vi "Vision Processing.vi"(4 "error in (no error)":errorcluster) -> ()   [LabVIEW 2016]
doc: "This VI runs in parallel to other tasks. It gets images from the camera, processes them for color or shape and use that information to affect robot behavior."
uses:
  <vilib>/Rock Robotics/WPI/Camera/WPI_CameraImageSize.ctl
  Camera Settings.ctl
  38 Video Mode.ctl
  Robot Global Data.vi
  <vilib>/Rock Robotics/WPI/Camera/WPI_CameraWhite Balance Values.ctl
  <vilib>/Rock Robotics/WPI/Camera/WPI_CameraExposure Values.ctl
  <vilib>/Rock Robotics/WPI/Camera/WPI_CameraFrameRate.ctl
panel:
  out "Image":T1(plugin-control)
  in  "error in (no error) 2":errorcluster
  out "Array 2":errorcluster[](array[cluster])
  in  "Image Size 2":T2=enum."320x240"
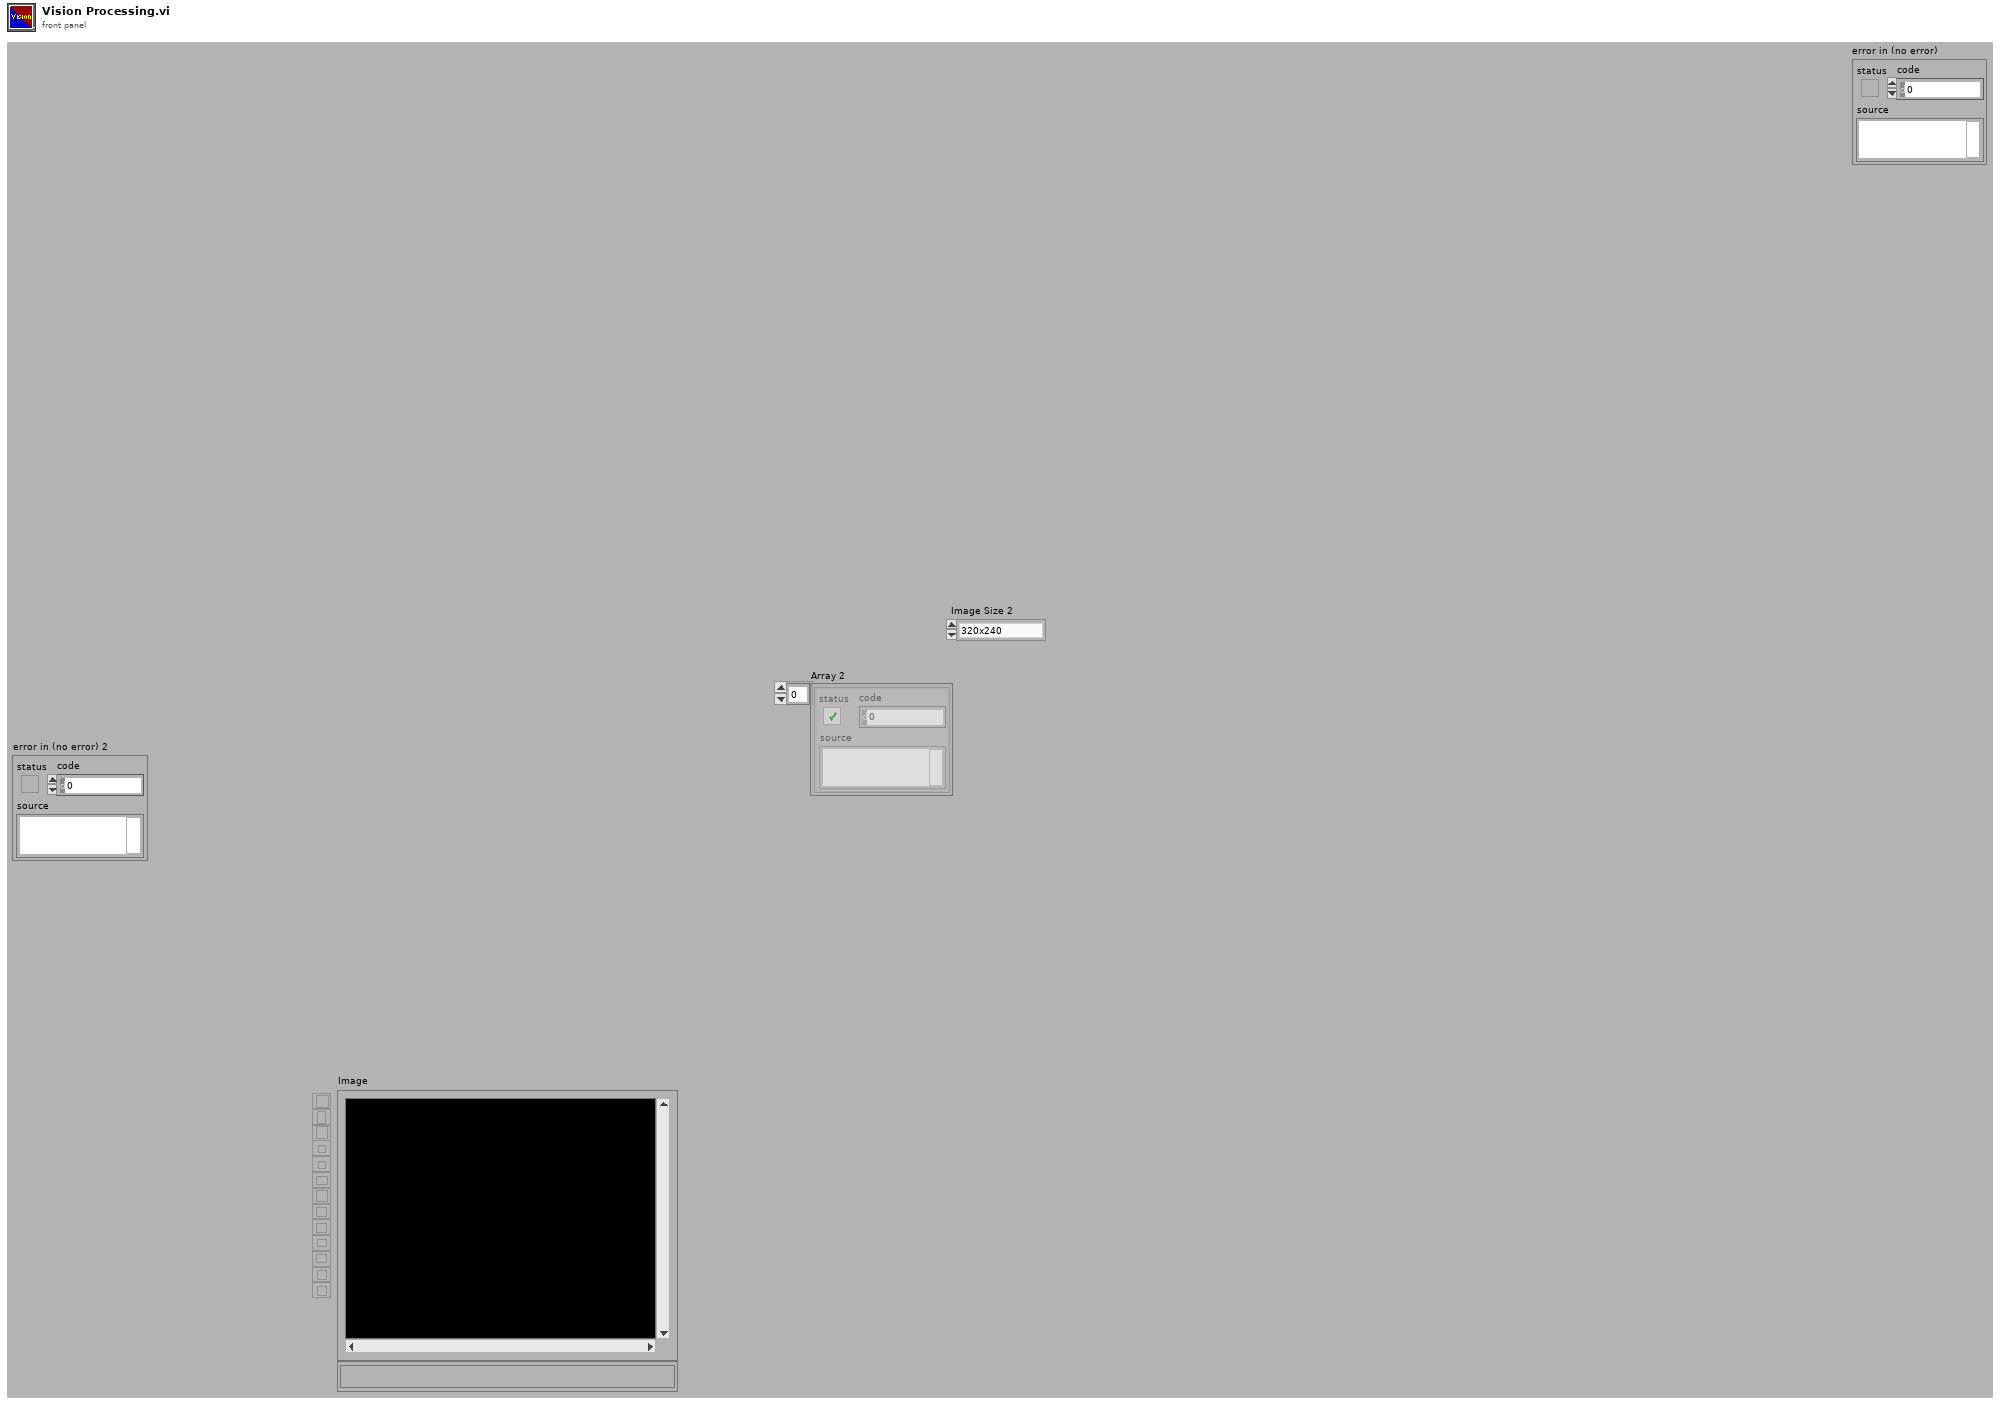
[diagram p1: front panel]
types:
  T1 = typedef "IMAQ Image.ctl" = refnum<image>
  T2 = typedef "WPI_CameraImageSize.ctl" = enum16{"640x480", "320x240", "160x120", "Custom"}
  T3 = typedef "Camera Settings.ctl" = cluster{"VideoMode":T4, "Brightness":i64, "Sharpness":i64, "White Balance":i64, "Saturation":i64, "Exposure":i64}
  T4 = typedef "38 Video Mode.ctl" = u32
  T5 = typedef "WPI_CameraFrameRate.ctl" = u32
  T6 = typedef "WPI_CameraExposure Values.ctl" = enum16{"Auto", "Flicker-free 50 Hz", "Flicker-free 60 Hz", "Hold current", "Custom"}
  T7 = typedef "WPI_CameraWhite Balance Values.ctl" = enum16{"Auto", "Fixed indoor", "Fixed outdoor 1", "Fixed outdoor 2", "Fixed fluorescent 1", "Fixed fluorescent 2", "Hold current", "Custom"}
  T8 = typedef "Image Type" = u32
  T9 = typedef "WPI_CameraDevRef.ctl" = cluster{"Camera Address":string, "CameraStatus":errorcluster}
  T10 = typedef "TCP Port Control.ctl" = cluster{"TCP Ports":cluster{"listener ID":refnum<k5>, "port":u16}[], "semaphore":T11, "occurrence":refnum<k4>, "Listener":refnum<data-value>}
  T11 = typedef "Semaphore RefNum" = refnum<k1>
  T12 = typedef "IMAQdx.ctl" = refnum<k21>
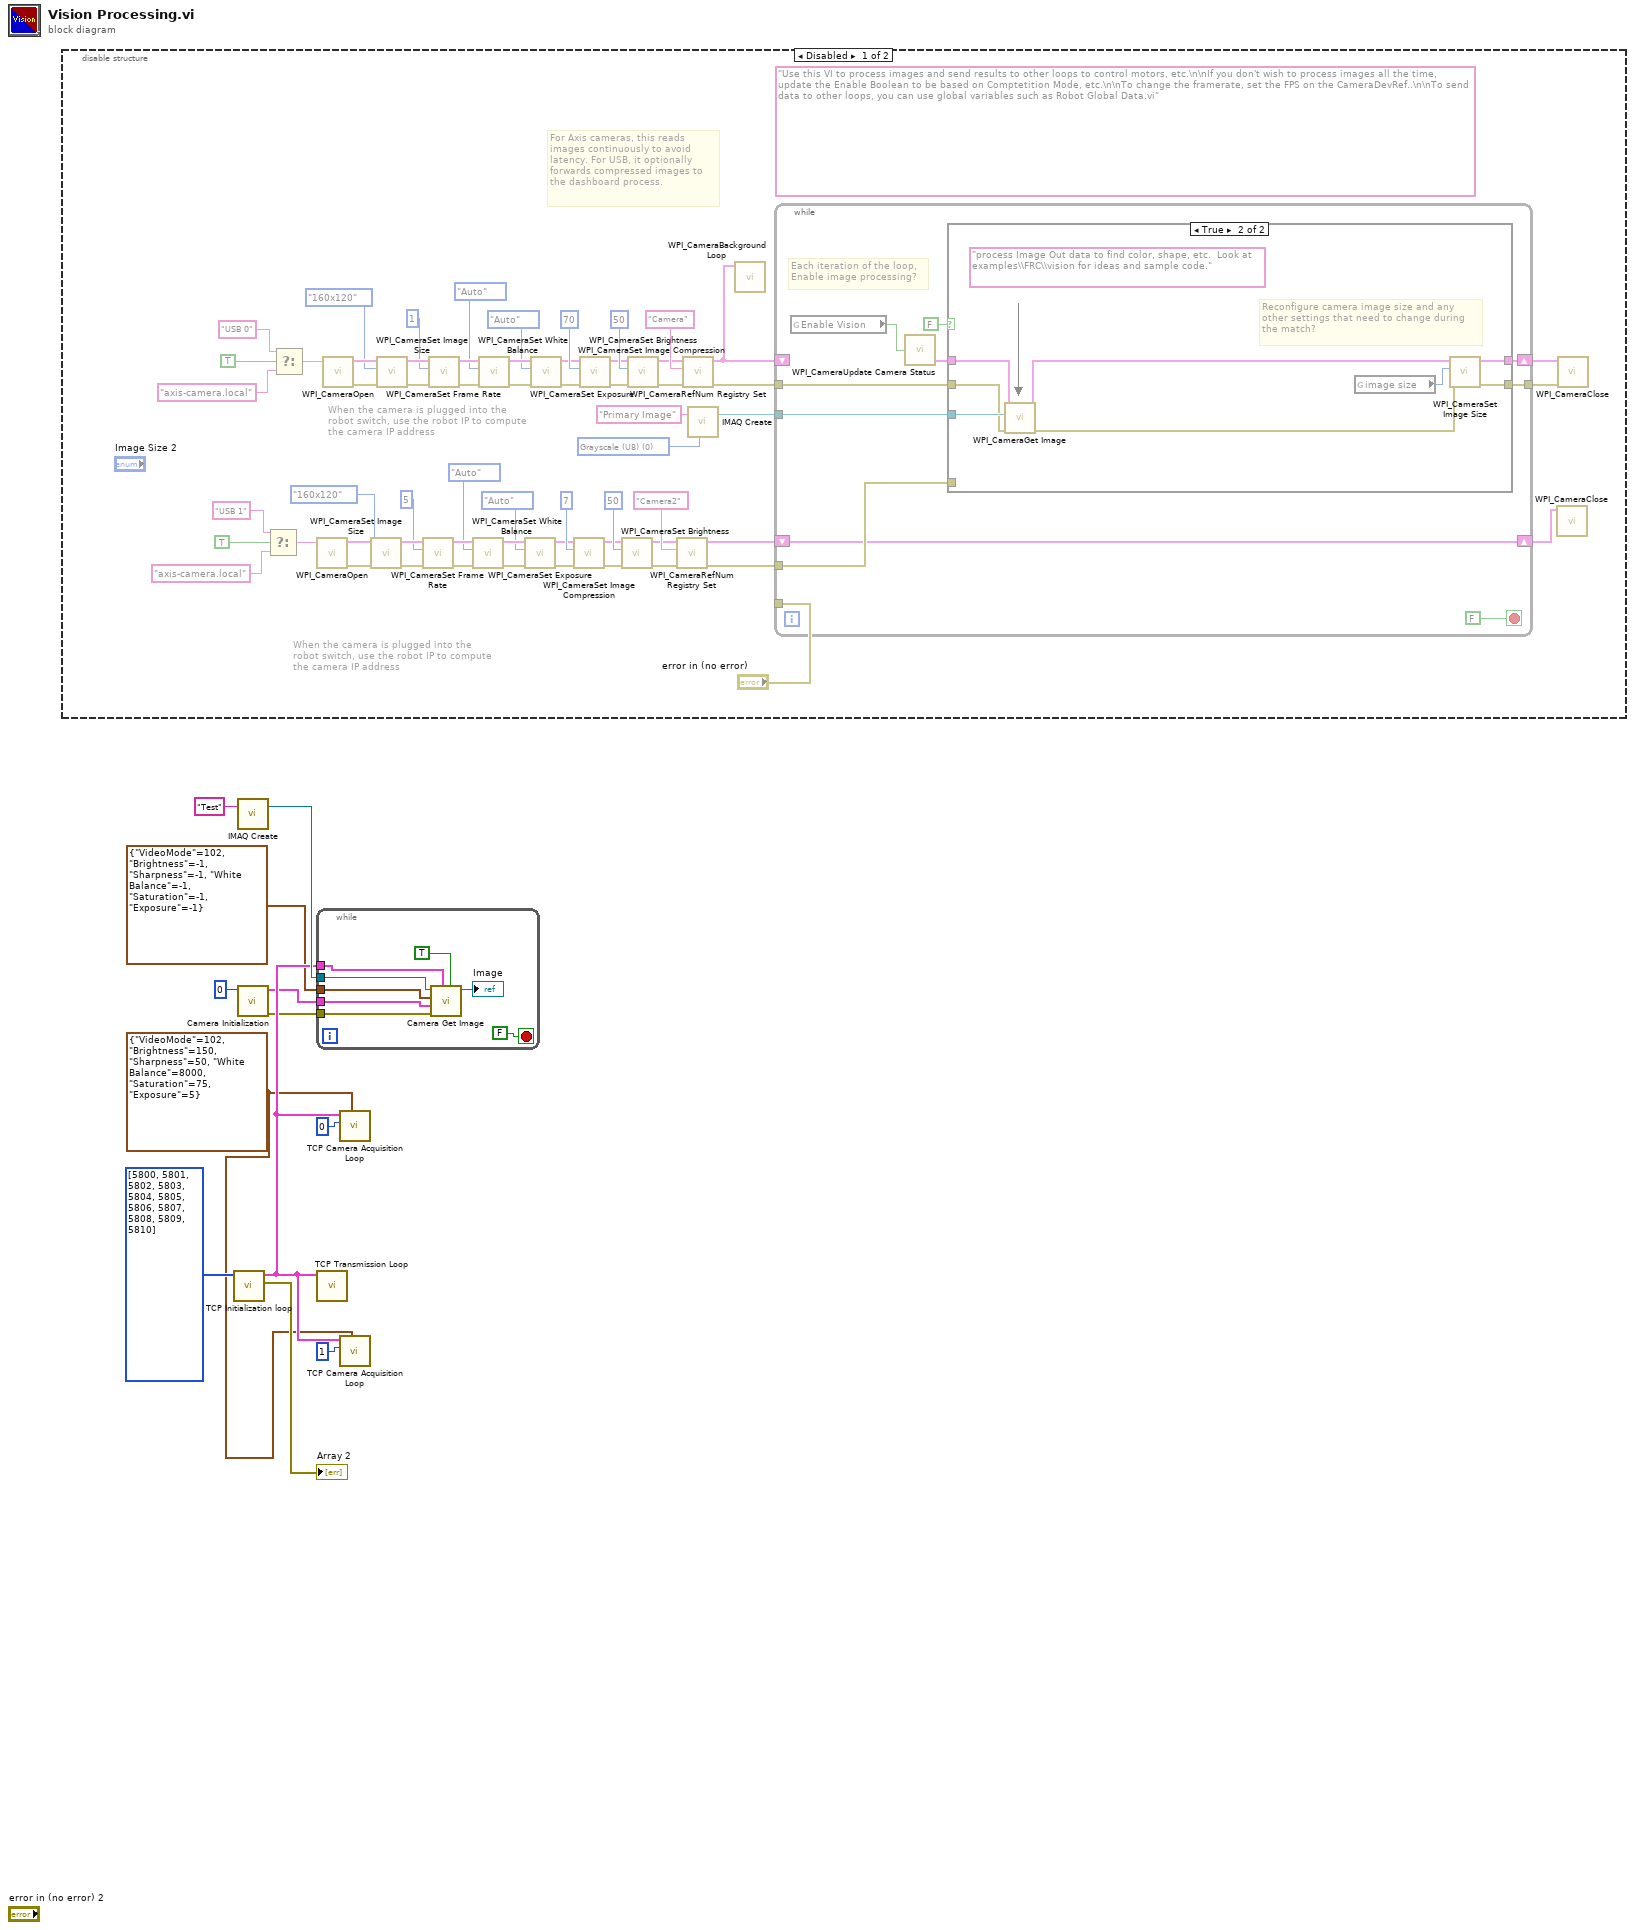
[diagram p0: block diagram]
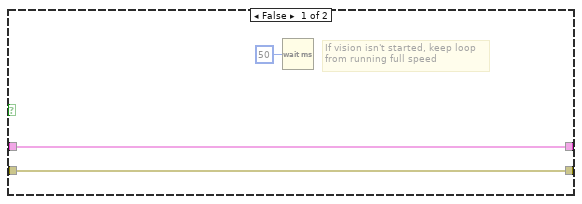
[diagram p2: hidden frame]
diagram:
  w1 = T3 {"VideoMode"=102, "Brightness"=150, "Sharpness"=50, "White Balance"=8000, "Saturation"=75, "Exposure"=5} ("Camera Controls")
  n1 = disable-structure shown="Disabled" {
    frame Disabled {
      (unwired) "Use this VI to process images and send results to other loops to control motors, etc.\n\nIf you don't wish to process images all the time, update the Enable Boolean to be based on Comptetition Mode, etc.\n\nTo change the framerate, set the FPS on the CameraDevRef..\n\nTo send data to other loops, you can use global variables such as Robot Global Data.vi"
      w73 = T8 0 items=["Grayscale (U8)", "Grayscale (I16)", "Grayscale (SGL)", "Complex (CSG)", "RGB (U32)", "HSL (U32)", "RGB (U64)"] ("Image Type")
      # "When the camera is plugged into the\nrobot switch, use the robot IP to compute\nthe camera IP address"
      # "When the camera is plugged into the\nrobot switch, use the robot IP to compute\nthe camera IP address"
      # "For Axis cameras, this reads\nimages continuously to avoid\nlatency. For USB, it optionally\nforwards compressed images to\nthe dashboard process."
      n2 = Select(t="USB 1" ("format string"), s=TRUE ("dot notation? (F)"), f="axis-camera.local" ("format string")) -> (s? t:f=w20:string)
      n3 = Select(t="USB 0" ("format string"), s=TRUE ("dot notation? (F)"), f="axis-camera.local" ("format string")) -> (s? t:f=w44:string)
      n4 = call <vilib>:"WPI_CameraOpen.vi"("Camera Address"=w20) -> ("error out"=w33:errorcluster, "CameraDevRef"=w34:T9)  [unwired: 1 in, 8 out]
      n5 = call <vilib>:"WPI_CameraOpen.vi"("Camera Address"=w44) -> ("error out"=w61:errorcluster, "CameraDevRef"=w62:T9)  [unwired: 1 in, 8 out]
      n6 = call <vilib>:"WPI_CameraSet Image Size.vi"("error in (no error)"=w33, "Image Size"=WPI_CameraImageSize."160x120", "CameraDevRef"=w34) -> ("error out"=w32:errorcluster, "CameraDevRef Out"=w35:T9)  [unwired: 1 in, 6 out]
      n7 = call <vilib>:"WPI_CameraSet Image Size.vi"("error in (no error)"=w61, "Image Size"=WPI_CameraImageSize."160x120", "CameraDevRef"=w62) -> ("error out"=w60:errorcluster, "CameraDevRef Out"=w63:T9)  [unwired: 1 in, 6 out]
      n8 = call <vilib>:"WPI_CameraSet Frame Rate.vi"("error in (no error)"=w32, "Frame Rate (fps)"=T5 5, "CameraDevRef"=w35) -> ("error out"=w31:errorcluster, "CameraDevRef Out"=w37:T9)  [unwired: 7 out]
      n9 = call <vilib>:"WPI_CameraSet Frame Rate.vi"("error in (no error)"=w60, "Frame Rate (fps)"=T5 1, "CameraDevRef"=w63) -> ("error out"=w59:errorcluster, "CameraDevRef Out"=w65:T9)  [unwired: 7 out]
      n10 = call <vilib>:"WPI_CameraSet White Balance.vi"("error in (no error)"=w31, "White Balance"=WPI_CameraWhite_Balance_Values."Auto", "CameraDevRef"=w37) -> ("error out"=w30:errorcluster, "CameraDevRef Out"=w36:T9)  [unwired: 1 in, 6 out]
      n11 = call <vilib>:"WPI_CameraSet White Balance.vi"("error in (no error)"=w59, "White Balance"=WPI_CameraWhite_Balance_Values."Auto", "CameraDevRef"=w65) -> ("error out"=w58:errorcluster, "CameraDevRef Out"=w64:T9)  [unwired: 1 in, 6 out]
      n12 = call <vilib>:"WPI_CameraSet Exposure.vi"("error in (no error)"=w30, "Exposure"=WPI_CameraExposure_Values."Auto", "CameraDevRef"=w36) -> ("error out"=w29:errorcluster, "CameraDevRef Out"=w39:T9)  [unwired: 1 in, 6 out]
      n13 = call <vilib>:"WPI_CameraSet Exposure.vi"("error in (no error)"=w58, "Exposure"=WPI_CameraExposure_Values."Auto", "CameraDevRef"=w64) -> ("error out"=w57:errorcluster, "CameraDevRef Out"=w67:T9)  [unwired: 1 in, 6 out]
      n14 = call <vilib>:"WPI_CameraSet Image Compression.vi"("error in (no error)"=w29, "Compression"=7, "CameraDevRef"=w39) -> ("error out"=w28:errorcluster, "CameraDevRef Out"=w38:T9)  [unwired: 7 out]
      n15 = call <vilib>:"WPI_CameraSet Image Compression.vi"("error in (no error)"=w57, "Compression"=70, "CameraDevRef"=w67) -> ("error out"=w56:errorcluster, "CameraDevRef Out"=w66:T9)  [unwired: 7 out]
      n16 = call <vilib>:"WPI_CameraSet Brightness.vi"("error in (no error)"=w28, "Brightness"=50, "CameraDevRef"=w38) -> ("error out"=w26:errorcluster, "CameraDevRef Out"=w27:T9)  [unwired: 7 out]
      n17 = call <vilib>:"WPI_CameraSet Brightness.vi"("error in (no error)"=w56, "Brightness"=50, "CameraDevRef"=w66) -> ("error out"=w54:errorcluster, "CameraDevRef Out"=w55:T9)  [unwired: 7 out]
      n18 = call <vilib>:"WPI_CameraRefNum Registry Set.vi"("error in (no error)"=w26, "refnum name"="Camera2", "CameraDevRef"=w27) -> ("error out"=w14:errorcluster, "CameraDevRef"=w13:T9)  [unwired: 1 in, 6 out]
      n19 = call <vilib>:"WPI_CameraRefNum Registry Set.vi"("error in (no error)"=w54, "refnum name"="Camera", "CameraDevRef"=w55) -> ("error out"=w16:errorcluster, "CameraDevRef"=w50:T9)  [unwired: 1 in, 6 out]
      n20 = call "IMAQ Create"("Image Name"="Primary Image", "Image Type"=w73) -> ("New Image"=w71:T1)  [unwired: 2 in, 2 out]
      n21 = call <vilib>:"WPI_CameraBackground Loop.vi"("CameraDevRef"=w50) -> ()  [unwired: 11 in]
      n22 = while {
        shift-right: [w82] -> w48
        shift-left: w50 -> [_]
        tunnel: w71 -> [w81]
        tunnel: "error in (no error)" -> [_]
        tunnel: w16 -> [w78]
        tunnel: [w77] -> w15
        tunnel: w14 -> [w76]
        shift-right: [w74] -> w18
        shift-left: w13 -> [w74]
        stop <- FALSE stop-if-true
        # "Each iteration of the loop,\nEnable image processing?"
        n23 = global read "Robot Global Data.vi" "Enable Vision"() -> (w79:bool)
        n24 = call <vilib>:"WPI_CameraUpdate Camera Status.vi"("Enable Vision"=w79) -> ("CameraDevRef Out"=w80:T9)  [unwired: 4 in]
        n25 = case shown="True" FALSE {
          tunnel: w81 -> [_ w93]
          tunnel: [w86 w94] -> w82
          tunnel: w80 -> [w86 w91]
          tunnel: w78 -> [w84 w89]
          tunnel: [w84 w87] -> w77
          tunnel: w76 -> [_ _]
          frame False {
            # "If vision isn't started, keep loop\nfrom running full speed"
            n26 = Wait (ms)(milliseconds to wait=u32 50) -> ()  [unwired: 1 out]
          }
          frame True {
            (unwired) "process Image Out data to find color, shape, etc.  Look at examples\\FRC\\vision for ideas and sample code."
            # "Reconfigure camera image size and any\nother settings that need to change during\nthe match?"
            n27 = call <vilib>:"WPI_CameraGet Image.vi"("error in (no error)"=w89, "Image"=w93, "CameraDevRef"=w91) -> ("error out"=w88:errorcluster, "CameraDevRef Out"=w90:T9)  [unwired: 7 out]
            n28 = global read "Robot Global Data.vi" "image size"() -> (w92:T2)
            n29 = call <vilib>:"WPI_CameraSet Image Size.vi"("error in (no error)"=w88, "Image Size"=w92, "CameraDevRef"=w90) -> ("error out"=w87:errorcluster, "CameraDevRef Out"=w94:T9)  [unwired: 1 in, 6 out]
          }
        }
      }
      n30 = call <vilib>:"WPI_CameraClose.vi"("CameraDevRef"=w18) -> ()  [unwired: 1 in, 10 out]
      n31 = call <vilib>:"WPI_CameraClose.vi"("error in (no error)"=w15, "CameraDevRef"=w48) -> ()  [unwired: 10 out]
    }
    frame Enabled {
    }
  }
  n32 = call "TCP Initialization loop.vi"("TCP Port Listen List"=u16[] [5800, 5801, 5802, 5803, 5804, 5805, 5806, 5807, 5808, 5809, 5810]) -> ("Array out"=→"Array 2":errorcluster[], "output cluster"=w7:T10)  [unwired: 9 in]
  n33 = call "IMAQ Create"("Image Name"="Test") -> ("New Image"=w9:T1)  [unwired: 4 in, 1 out]
  n34 = call "Camera Initialization.vi"("Camera Number"=0) -> ("error out"=w3:errorcluster, "Cluster"=w6:cluster{"Session Out":T12, "Camera Number":i32})  [unwired: 9 in]
  n35 = while {
    tunnel: w9 -> [w101]
    tunnel: w7 -> [w100]
    tunnel: w6 -> [w99]
    tunnel: T3 {"VideoMode"=102, "Brightness"=-1, "Sharpness"=-1, "White Balance"=-1, "Saturation"=-1, "Exposure"=-1} ("Camera Controls") -> [w98]
    tunnel: w3 -> [w97]
    stop <- FALSE stop-if-true
    n36 = call "Camera Get Image.vi"("Xmit"=TRUE, "Network Data"=w100, "error in (no error)"=w97, "Camera Cluster"=w99, "Camera Controls"=w98, "Refnum in"=w101) -> ("Refnum out"=→"Image":T1)  [unwired: 5 in]
  }
  n37 = call "TCP Transmission Loop.vi"("output cluster"=w7) -> ()  [unwired: 11 in]
  n38 = call "TCP Camera Acquisition Loop.vi"("Camera Controls"=w1, "Camera Number"=0, "Transmission Cluster"=w7) -> ()  [unwired: 9 in]
  n39 = call "TCP Camera Acquisition Loop.vi"("Camera Controls"=w1, "Camera Number"=1, "Transmission Cluster"=w7) -> ()  [unwired: 9 in]
